vi "BristolFirstProg.vi"() -> ()   [LabVIEW 2012]
uses:
  00424-2-00 621 customer CD/Programming Interface/x32/CLDevIFace.dll
panel:
  out "return type":dbl
  in  "comm port":i32
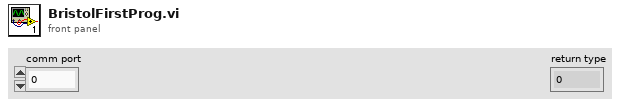
[diagram p1: front panel]
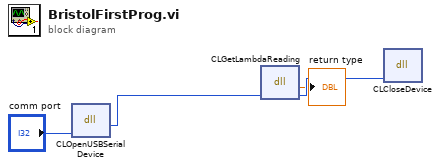
[diagram p0: block diagram]
diagram:
  n1 = dll-call lib="C:/Users/Lab/Desktop/Bristol wavemeter 621/00424-2-00 621 customer CD/Programming Interface/x32/CLDevIface.dll" fn="CLOpenUSBSerialDevice"("comm port"="comm port") -> ("return type"=w3:i32)  [unwired: 4 in, 2 out]
  n2 = dll-call lib="C:/Users/Lab/Desktop/Bristol wavemeter 621/00424-2-00 621 customer CD/Programming Interface/x32/CLDevIface.dll" fn="CLGetLambdaReading"("devHandle"=w3) -> ("return type"=→"return type":dbl, "devHandle"=w2:i32)  [unwired: 3 in, 2 out]
  n3 = dll-call lib="C:/Users/Lab/Desktop/Bristol wavemeter 621/00424-2-00 621 customer CD/Programming Interface/x32/CLDevIFace.dll" fn="CLCloseDevice"("comm port"=w2) -> ()  [unwired: 5 in, 2 out]
